vi "ColorDetect_V2.vi"(0 "new picture":picture, 5 "Color 1 Lower":u32(colorbox), 7 "Color 1 Upper":u32(colorbox), 11 "error in (no error)":errorcluster) -> (4 "out picture":picture, 6 "image":u8[][](array[numeric]), 8 "found (X,Y,R)":u32[][](array[numeric]), 15 "error out":errorcluster)   [LabVIEW 2014, in "QwaveSys RPi Training Library.lvlib"]
uses:
  <vilib>/Q-Wave Systems/QwaveSys RPi Package 2.0/Addons/QwaveSys RPi Training Library.lvlib
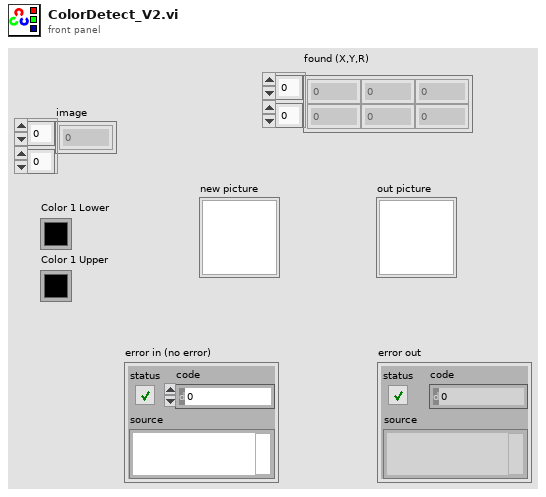
[diagram p1: front panel]
types:
  T1 = cluster{"Width":u16, "Style":enum32{"Solid", "Dash", "Dot", "DashDot", "DashDotDot"}}
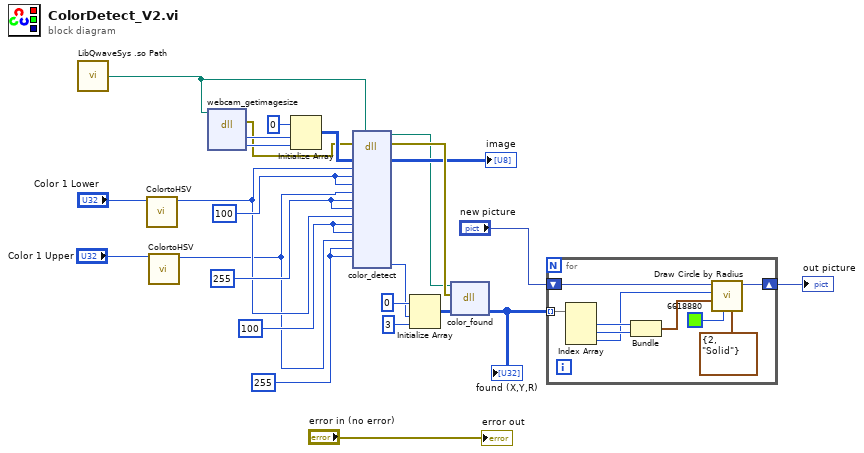
[diagram p0: block diagram]
diagram:
  w9 = u8 100
  w8 = u8 255
  w10 = u8 255
  w11 = u8 100
  n1 = call <vilib>:"LibQwaveSys .so Path.vi"() -> ("Lib QwaveSys .so Path"=w2:path)  [unwired: 5 in]
  n2 = call <vilib>:"ColortoHSV.vi"("Color Box"="Color 1 Lower") -> ("Hue (0-180)"=w7:u8)  [unwired: 7 in, 3 out]
  n3 = call <vilib>:"ColortoHSV.vi"("Color Box"="Color 1 Upper") -> ("Hue (0-180)"=w6:u8)  [unwired: 7 in, 3 out]
  n4 = dll-call lib="libqwavesys.so" fn="webcam_getimagesize"(path in=w2) -> (error out=w3:errorcluster, "rows"=w24:i32, "cols"=w25:i32)  [unwired: 5 in, 1 out]
  n5 = Initialize Array(u8 0 ("element"), w24, w25) -> (w23:u8[][])
  n6 = dll-call lib="libqwavesys.so" fn="color_detect"(path in=w2, error in=w3, "image"=w23, "Alower_h"=w7, "Alower_s"=w11, "Alower_v"=w11, "Aupper_h"=w6, "Aupper_s"=w10, "Aupper_v"=w10, "Blower_h"=w7, "Blower_s"=w9, "Blower_v"=w9, "Bupper_h"=w6, "Bupper_s"=w8, "Bupper_v"=w8) -> (path out=w1:path, error out=w15:errorcluster, "image"=→"image":u8[][], "found"=w14:i32)  [unwired: 15 in]
  n7 = Initialize Array "Initialize Array"(u32 0 ("element"), w14, 3 ("dimension size")) -> (w19:u32[][])
  n8 = dll-call lib="libqwavesys.so" fn="color_found"(path in=w1, error in=w15, "found"=w19) -> ("found"=w17:u32[][])  [unwired: 2 in, 2 out]
  "found (X,Y,R)" <- w17
  n9 = for {
    tunnel: w17 -> [w32] mode=indexing
    shift-right: [w26] -> w4
    shift-left: "new picture" -> [w27]
    n10 = Index Array(array=w32) -> (element #1=w31:u32, element #2=w30:u32, element #3=w29:u32)  [unwired: 3 in]
    n11 = Bundle(w31, w30) -> (w34:cluster{u32, u32})  [unwired: 1 in]
    n12 = call <vilib>:"Draw Circle by Radius.vi"("pen"=T1 {"Width"=2, "Style"=enum."Solid"}, "color(black)"=u32 6618880, "pixel center"=w34, "radius"=w29, "picture"=w27) -> ("new picture"=w26:picture)  [unwired: 6 in]
  }
  "out picture" <- w4
  "error out" <- "error in (no error)"
